vi "SetReg.vi"(2 "SetReg":i32 format="%.0b", 3 "Register":u32, 4 "Controller ID":u32) -> (0 "Err Msg":string, 1 "err":bool)   [LabVIEW 2011]
uses:
  Windows/System32/CTCEmcorev2.dll
panel:
  in  "stop":bool
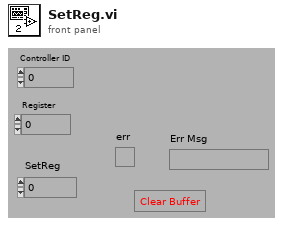
[diagram p1: front panel]
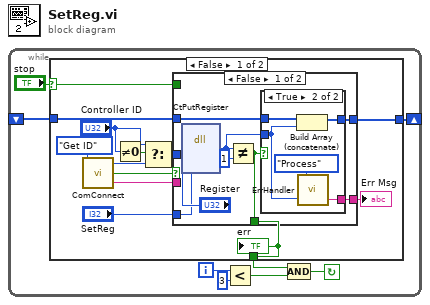
[diagram p0: block diagram]
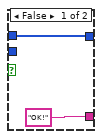
[diagram p2: hidden frame]
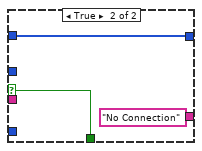
[diagram p3: hidden frame]
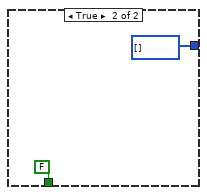
[diagram p4: hidden frame]
diagram:
  n1 = while {
    shift-left: _ -> [w6]
    shift-right: [w7] -> _
    i -> [w2]
    stop <- w5 continue-if-true
    n2 = case shown="False" "stop" {
      selector: "stop" -> [w14 _]
      tunnel: [w16 i32[] []] -> w7
      tunnel: w6 -> [w15 _]
      tunnel: [w13 FALSE] -> w4
      frame False {
        n3 = call "ComConnect.vi"("Action"=enum16{"Open", "Get ID", "Close"}."Get ID") -> ("ConnectID"=w12:u32, "err"=w20:bool, "Err Msg"=w19:string)
        n4 = Not Equal To 0?(x="Controller ID") -> (x != 0?=w10:bool)
        n5 = Select(t="Controller ID", s=w10, f=w12) -> (s? t:f=w11:u32)
        n6 = case shown="False" w20 {
          selector: w20 -> [_ w40]
          tunnel: [w28 "No Connection"] -> w18
          tunnel: w19 -> [_ _]
          tunnel: [w23 w40] -> w13
          tunnel: w11 -> [w22 _]
          tunnel: "SetReg" -> [w27 _]
          tunnel: [w26 w39] -> w16
          tunnel: w15 -> [w24 w39]
          tunnel: w14 -> [_ _]
          frame False {
            n7 = dll-call lib="C:/Windows/System32/CtcEmcorev2.dll" fn="CtPutRegister"("ConnectID"=w22, "Register"="Register", "pValue"=w27) -> (w25:u32)  [unwired: 6 in, 2 out]
            n8 = Not Equal?(x=w25, y=u32 1) -> (x != y?=w23:bool)
            n9 = case shown="True" w23 {
              tunnel: ["OK!" w37] -> w28
              tunnel: [w32 w36] -> w26
              tunnel: w25 -> [_ w33]
              tunnel: w24 -> [w32 w35]
              frame False {
              }
              frame True {
                n10 = Build Array (concatenate)(w35, w33) -> (w36:u32[])
                n11 = call "ErrHandler.vi"("Err Code"=w33, "Action"=enum16{"Init", "Process"}."Process") -> ("Err Msg"=w37:string)
              }
            }
          }
          frame True {
          }
        }
        "err" <- w13
        "Err Msg" <- w18
      }
      frame True {
      }
    }
    n12 = Less?(x=w2, y=3) -> (x < y?=w3:bool)
    n13 = Compound Arithmetic op=AND(w4, w3) -> (w5:bool)
  }
